vi "GetImageAsPixmap.vi"(8 "error in (no error)":errorcluster, 10 "Get Image (-1: latest)":i32=-1, 11 "Camera":refnum<class "Camera.lvclass">) -> (0 "error out":errorcluster, 2 "pixmap":u32[][](array[numeric]), 3 "Camera out":refnum<class "Camera.lvclass">)   [LabVIEW 2015, in "Camera.lvclass"]
doc: "---------------------------------------------------------------\nJKI State Machine Objects™\nhttp://jki.net/state-machine-objects/\nCopyright (C) 2005-2015, JKI <info@jki.net>\nALL RIGHTS RESERVEDJKI State Machine Objects (SMO) 1.0.0.4\nJKI - JKI\nCopyright (c) 2015, JKI"
uses:
  Camera.lvclass
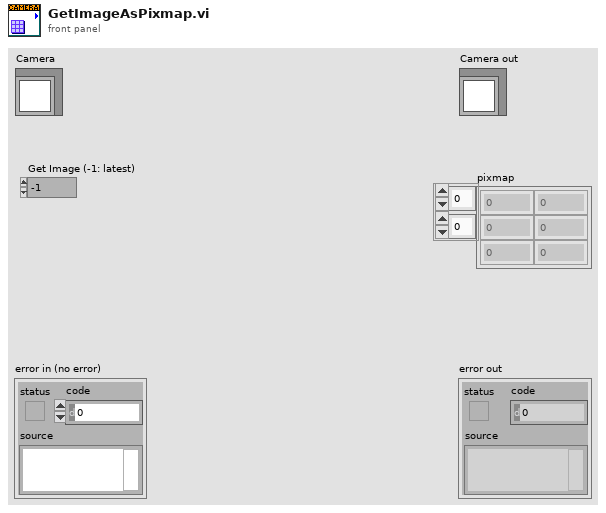
[diagram p1: front panel]
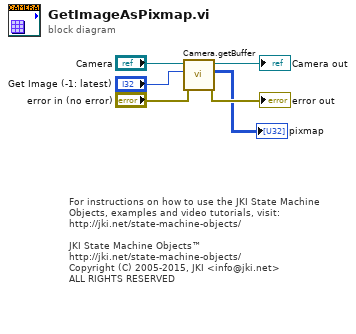
[diagram p0: block diagram]
diagram:
  # "For instructions on how to use the JKI State Machine Objects, examples and video tutorials, visit:\nhttp://jki.net/state-machine-objects/\n\nJKI State Machine Objects™\nhttp://jki.net/state-machine-objects/\nCopyright (C) 2005-2015, JKI <info@jki.net>\nALL RIGHTS RESERVED"
  n1 = call-dynamic "Camera.getBuffer.vi"("error in (no error)"="error in (no error)", "Get Image (-1: latest)"="Get Image (-1: latest)", "Camera in"="Camera") -> ("error out"=→"error out":errorcluster, "pixmap"=→"pixmap":u32[][], "Camera out"=→"Camera out":refnum<class "Camera.lvclass">)  [unwired: 6 in]
